vi "CMD_Object Command.vi"(8 "error in (no error)":errorcluster, 9 "Command":string, 10 "Object":string, 11 "Queue in":refnum<queue>) -> (0 "error out":errorcluster, 3 "Queue out":refnum<queue>)   [LabVIEW 2025]
uses:
  <vilib>/Handler Framework/Handler Framework.lvlib
  <vilib>/Handler Framework/CmdQueue/Enqueue Single.vi
panel:
  out "appended array":string[](array[string])
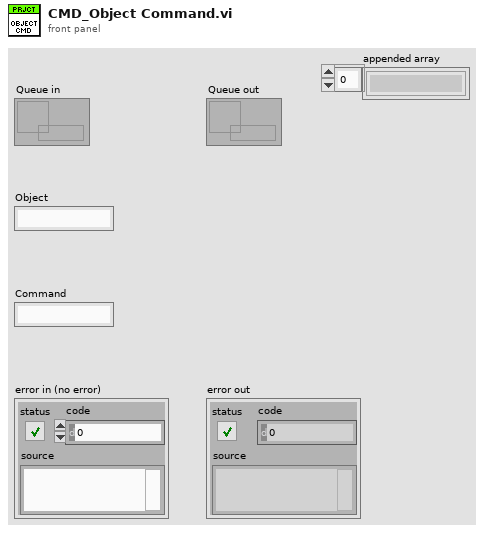
[diagram p1: front panel]
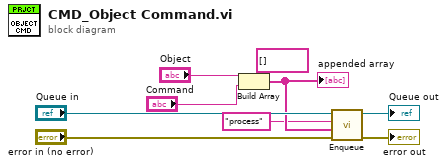
[diagram p0: block diagram]
diagram:
  (unwired) string[] [] ("appended array")
  n1 = Build Array("Object", "Command") -> (w6:string[])
  "appended array" <- w6
  n2 = call-poly <vilib>:"Enqueue.vi"("error in (no error)"="error in (no error)", "Value"=w6, "Command"="process", "CmdQueue in"="Queue in") -> ("error out"=→"error out":errorcluster, "CmdQueue out"=→"Queue out":refnum<queue>)  [unwired: 6 in]
